vi "Lettura 3 Proximity_fin excel .vi"() -> ()   [LabVIEW 2020]
uses:
  <vilib>/DAQmx/read.llb/DAQmx Read (Analog 1D Wfm NChan NSamp).vi
  <vilib>/Analysis/baseanly.llb/Mean (DBL).vi
  <vilib>/DAQmx/configure/timing.llb/DAQmx Timing (Sample Clock).vi
  <vilib>/DAQmx/miscellaneous.llb/DAQmx Fill In Error Info.vi
  <vilib>/Utility/file.llb/Write Delimited Spreadsheet (DBL).vi
  <vilib>/Analysis/NI_AALBase.lvlib
panel:
  in  "File Excel 3 Sensori":path
  in  "File txt Tensione 1":path
  out "Distanza 1":dbl[](graph)
  in  "File txt Distanza 1":path
  out "Media 3":dbl format="%0.2f"
  out "Deviazione Standard 3":dbl format="%0.2f"
  out "Massimo3":dbl
  out "Minimo 3":dbl
  in  "File txt Tensione 2":path
  out "Distanza 2":dbl[](graph)
  in  "File txt Distanza 2":path
  out "Media 2":dbl format="%0.2f"
  out "Deviazione Standard 2":dbl format="%0.2f"
  out "Massimo 2":dbl
  out "Minimo 2":dbl
  out "Segnale Proximity 1":dynamicdata(graph)
  out "Segnale Proximity 2":dynamicdata(graph)
  out "Minimo":dbl
  out "Massimo":dbl
  out "Deviazione Standard":dbl format="%0.2f"
  out "Media":dbl format="%0.2f"
  in  "File txt Distanza 3":path
  out "Distanza 3":dbl[](graph)
  out "Segnale Proximity 3":dynamicdata(graph)
  out "num campioni":dbl
  in  "File txt Tensione 3":path
  in  "SAVE":bool
  in  "Frequenza":dbl=5000.0 format="%0.2p"
  in  "Durata":dbl=0.1 format="%.2p"
  in  "STOP":bool
  out "current time":timestamp
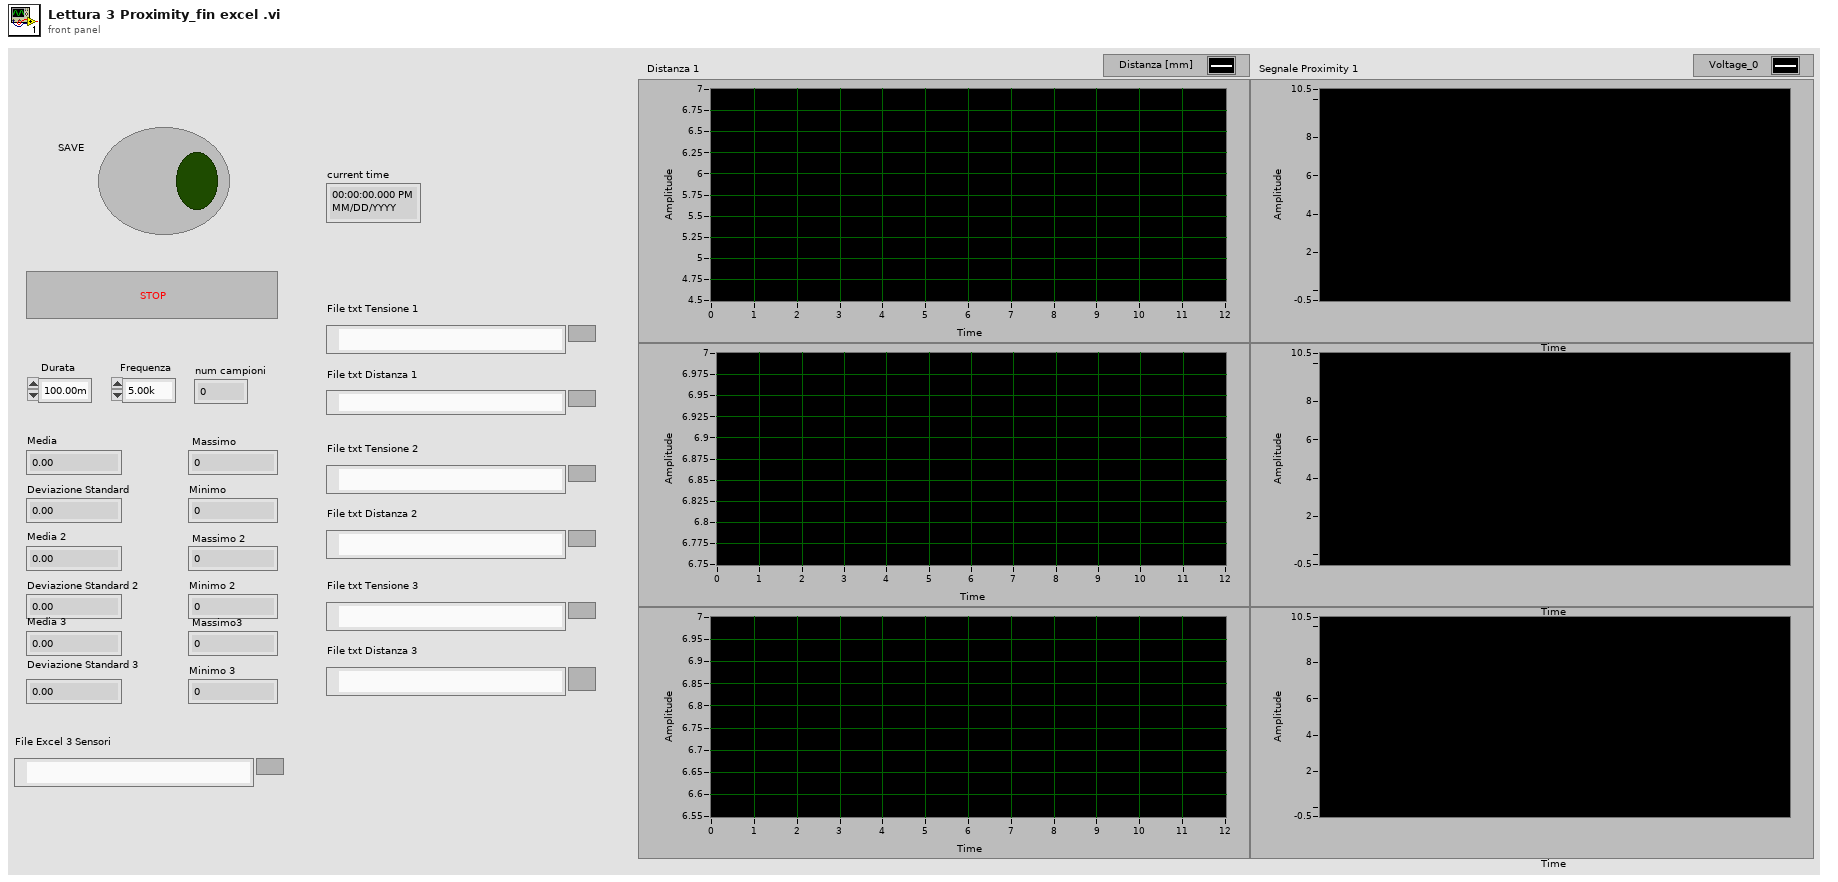
[diagram p1: front panel]
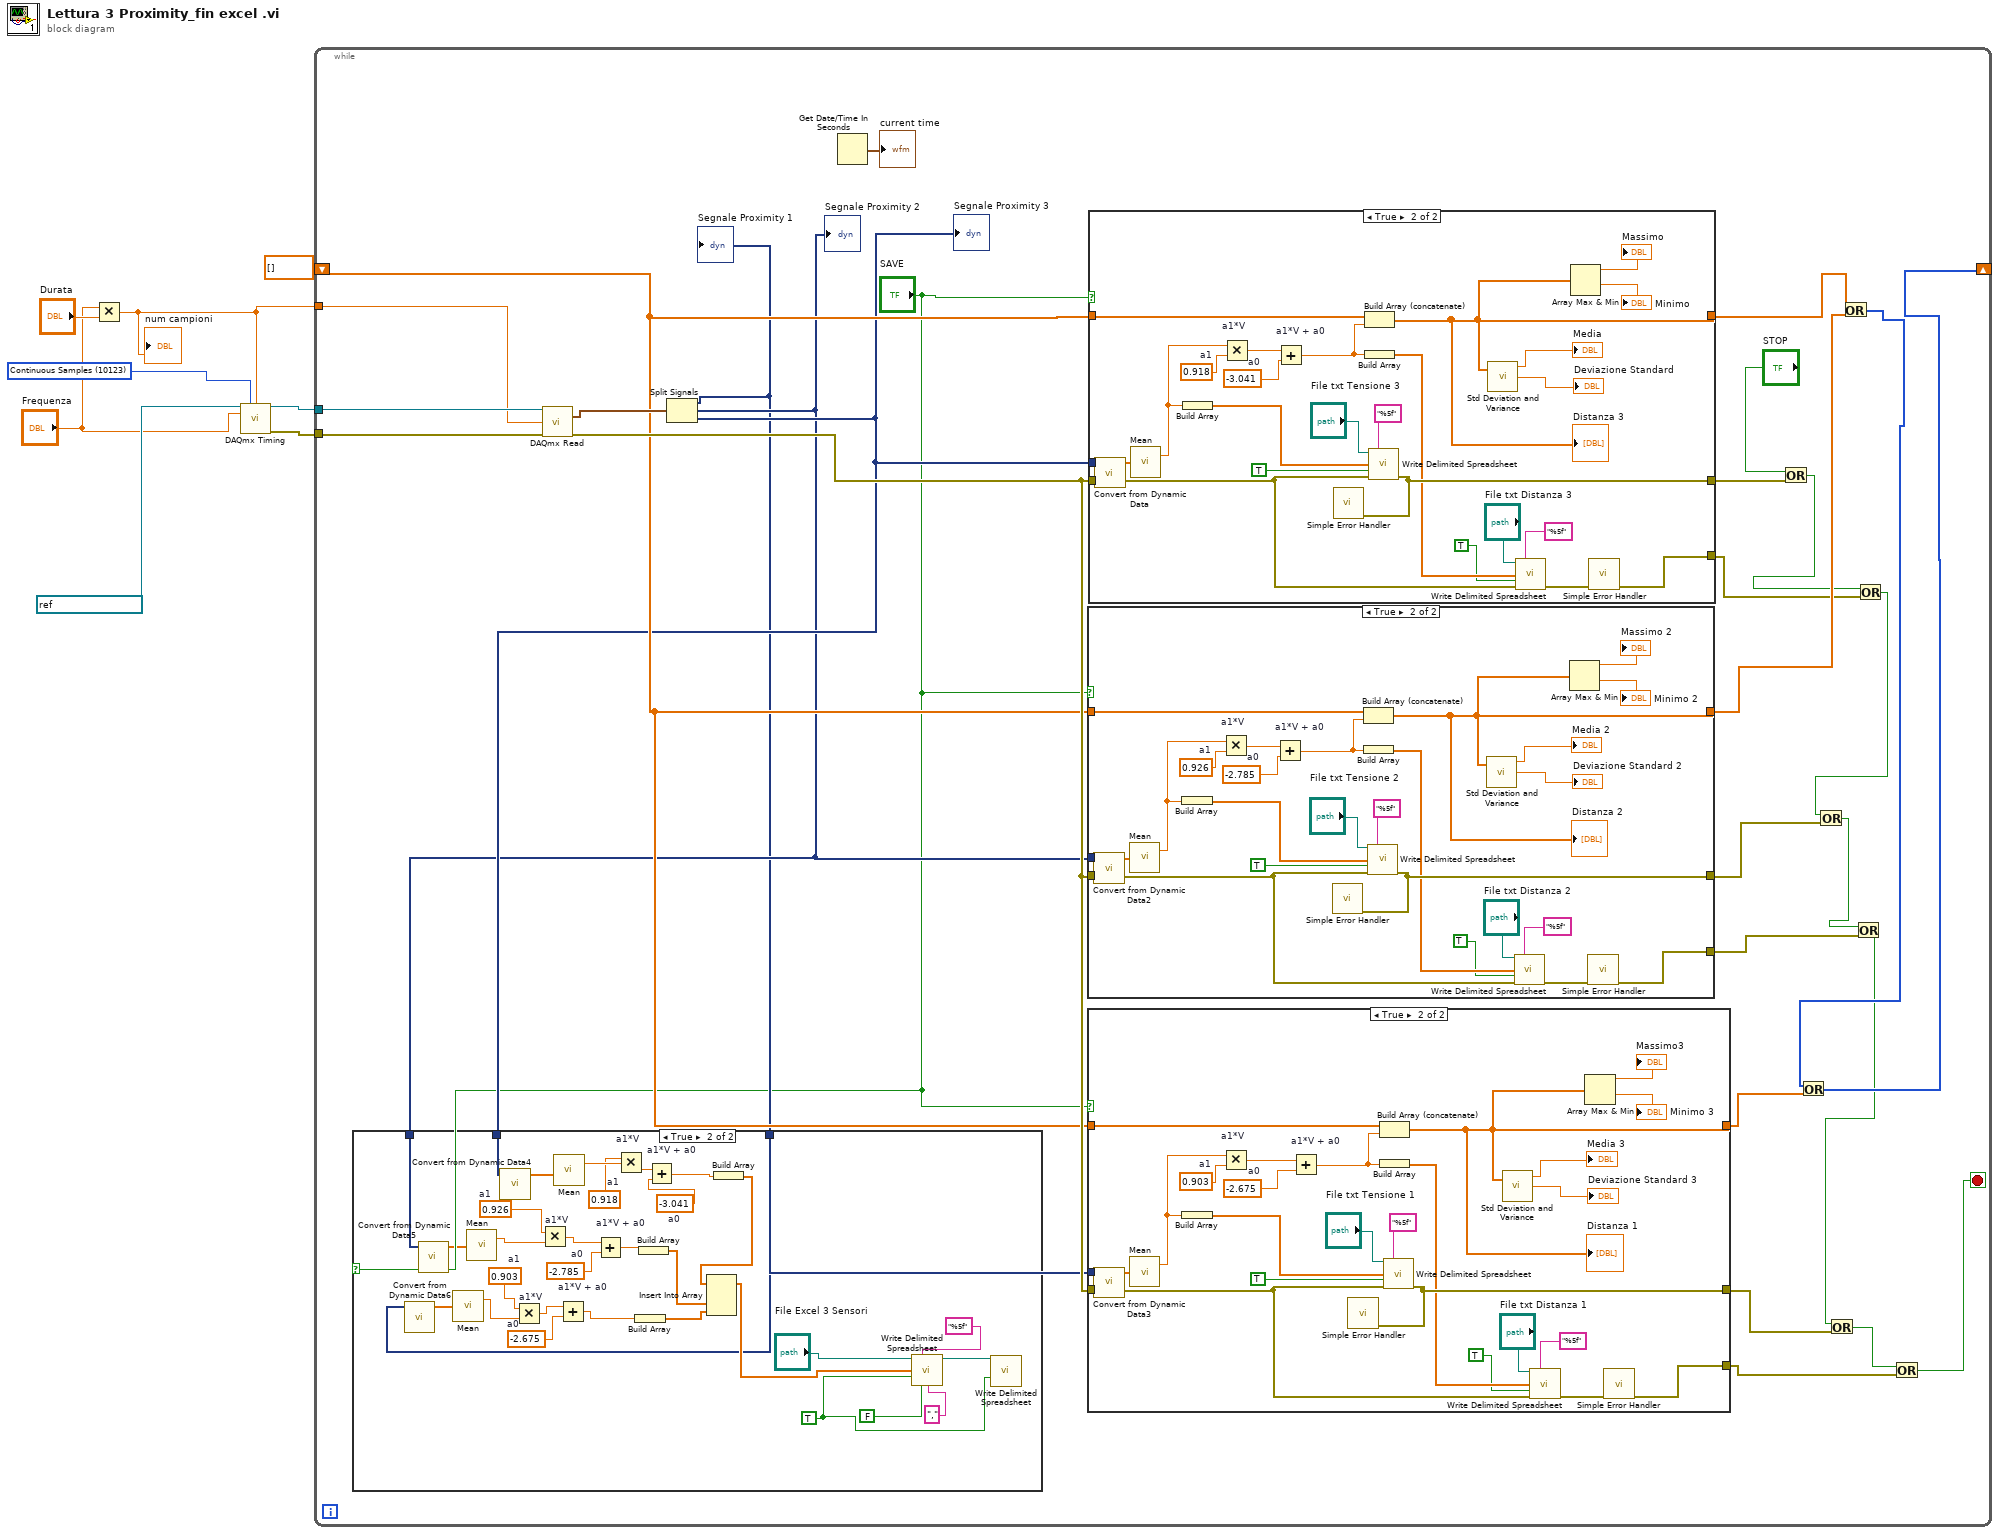
[diagram p0: block diagram]
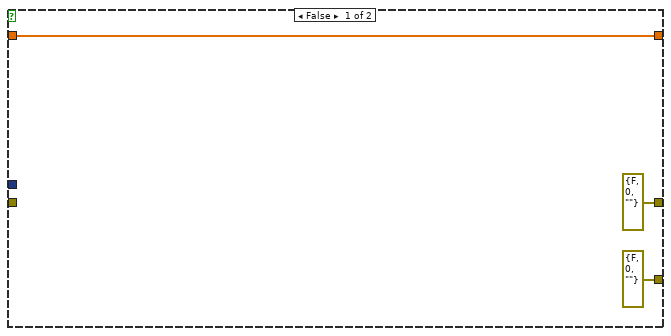
[diagram p3: hidden frame]
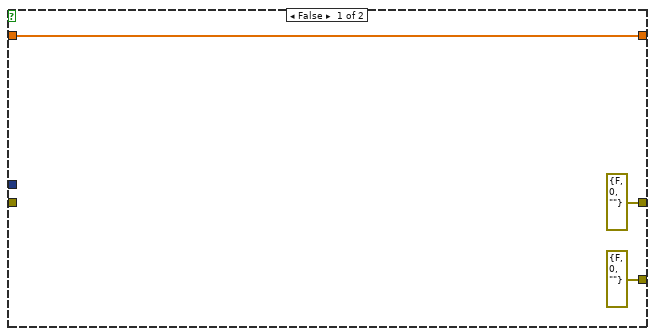
[diagram p4: hidden frame]
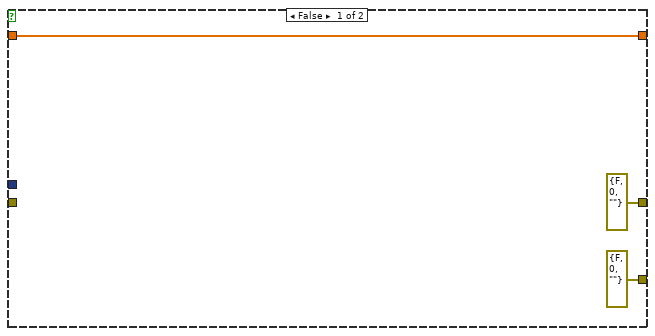
[diagram p5: hidden frame]
diagram:
  w4 = 10123 items=["Finite Samples"=10178, "Continuous Samples"=10123, "Hardware Timed Single Point"=12522] ("sample mode")
  n1 = Multiply(x="Frequenza", y="Durata") -> (x*y=w5:dbl)
  "num campioni" <- w5
  n2 = call-poly <vilib>:"DAQmx Timing.vi"("task/channels in"=refnum<k21> "MyVoltageTask", "sample mode"=w4, "samples per channel"=w5, "rate"="Frequenza") -> ("task out"=w8:refnum<k21>, "error out"=w3:errorcluster)  [unwired: 10 in]
  n3 = while {
    tunnel: w8 -> [w36]
    tunnel: w5 -> [w35]
    tunnel: w3 -> [w34]
    shift-right: [w23] -> _
    shift-left: dbl[] [] -> [w21]
    stop <- w13 stop-if-true
    n4 = call-poly <vilib>:"DAQmx Read.vi"("task/channels in"=w36, "number of samples per channel"=w35, "error in"=w34) -> ("data"=w32:waveform(dbl)[], "error out"=w22:errorcluster)  [unwired: 10 in, 1 out]
    n5 = Split Signals(w32) -> (w10:dynamicdata, w11:dynamicdata, w12:dynamicdata)  [unwired: 3 in]
    "Segnale Proximity 3" <- w12
    "Segnale Proximity 2" <- w11
    "Segnale Proximity 1" <- w10
    n6 = case shown="True" "SAVE" {
      tunnel: w12 -> [_ w63]
      tunnel: w11 -> [_ w54]
      tunnel: w10 -> [_ w62]
      frame False {
      }
      frame True {
        w40 = -2.675  # a0
        w43 = 0.903  # a1
        w41 = -2.785  # a0
        w45 = 0.926  # a1
        w46 = -3.041  # a0
        w47 = 0.918  # a1
        w38 = TRUE ("append to file? (new file:F)")
        n7 = call "Convert from Dynamic Data6"("Dynamic Data Type"=w62) -> ("Array"=w64:dbl[])  [unwired: 3 in]
        n8 = call "Convert from Dynamic Data5"("Dynamic Data Type"=w54) -> ("Array"=w53:dbl[])  [unwired: 3 in]
        n9 = call-poly <vilib>:"Mean.vi"("X"=w64) -> ("mean"=w49:dbl)  [unwired: 1 out]
        n10 = call-poly <vilib>:"Mean.vi"("X"=w53) -> ("mean"=w52:dbl)  [unwired: 1 out]
        n11 = call "Convert from Dynamic Data4"("Dynamic Data Type"=w63) -> ("Array"=w65:dbl[])  [unwired: 3 in]
        n12 = Multiply "a1*V"(x=w43, y=w49) -> (x*y=w44:dbl)
        n13 = Multiply "a1*V"(x=w45, y=w52) -> (x*y=w42:dbl)
        n14 = call-poly <vilib>:"Mean.vi"("X"=w65) -> ("mean"=w55:dbl)  [unwired: 1 out]
        n15 = Add "a1*V + a0"(x=w44, y=w40) -> (x+y=w48:dbl)
        n16 = Add "a1*V + a0"(x=w42, y=w41) -> (x+y=w51:dbl)
        n17 = Multiply "a1*V"(x=w47, y=w55) -> (x*y=w58:dbl)
        n18 = Build Array(w48) -> (w61:dbl[])
        n19 = Build Array(w51) -> (w50:dbl[])
        n20 = Add "a1*V + a0"(x=w58, y=w46) -> (x+y=w57:dbl)
        n21 = Build Array(w57) -> (w56:dbl[])
        n22 = Insert Into Array(array=w56, new element #1=w50, new element #2=w61) -> (w66:dbl[])  [unwired: 1 in]
        n23 = call-poly <vilib>:"Write Delimited Spreadsheet.vi"("file path (dialog if empty)"="File Excel 3 Sensori", "format (%.3f)"="%5f", "1D data"=w66, "append to file? (new file:F)"=w38, "transpose? (no:F)"=FALSE ("append to file? (new file:F)"), "delimiter (\\t)"="," ("format (%.3f)")) -> ("new file path (Not A Path if cancelled)"=w39:path)  [unwired: 8 in, 1 out]
        n24 = call-poly <vilib>:"Write Delimited Spreadsheet.vi"("file path (dialog if empty)"=w39, "append to file? (new file:F)"=w38) -> ()  [unwired: 12 in, 2 out]
      }
    }
    n25 = Get Date/Time In Seconds() -> (seconds since 1Jan1904=→"current time":timestamp)
    n26 = case shown="True" "SAVE" {
      tunnel: [errorcluster {"status"=FALSE, "code"=0, "source"=""} ("error IO") w123] -> w29
      tunnel: w11 -> [_ w122]
      tunnel: w22 -> [_ w115]
      tunnel: [w98 w103] -> w31
      tunnel: w21 -> [w98 w106]
      tunnel: [errorcluster {"status"=FALSE, "code"=0, "source"=""} ("error out") w113] -> w25
      frame False {
      }
      frame True {
        w108 = -2.785  # a0
        w109 = 0.926  # a1
        n27 = call "Convert from Dynamic Data2"("Dynamic Data Type"=w122) -> ("Array"=w100:dbl[])  [unwired: 3 in]
        n28 = call-poly <vilib>:"Mean.vi"("X"=w100) -> ("mean"=w110:dbl)  [unwired: 1 out]
        n29 = Build Array(w110) -> (w119:dbl[])
        n30 = Multiply "a1*V"(x=w110, y=w109) -> (x*y=w111:dbl)
        n31 = Add "a1*V + a0"(x=w111, y=w108) -> (x+y=w107:dbl)
        n32 = Build Array (concatenate)(w106, w107) -> (w103:dbl[])
        "Distanza 2" <- w103
        n33 = Build Array(w107) -> (w118:dbl[])
        n34 = call-poly <vilib>:"Write Delimited Spreadsheet.vi"("file path (dialog if empty)"="File txt Tensione 2", "format (%.3f)"="%5f", "1D data"=w119, "append to file? (new file:F)"=TRUE, "error in (no error)"=w115) -> ("error out"=w123:errorcluster)  [unwired: 9 in, 1 out]
        n35 = call <vilib>:"Simple Error Handler.vi"("error in (no error)"=w123) -> ()  [unwired: 4 in, 5 out]
        n36 = call <vilib>:"Std Deviation and Variance.vi"("X"=w103) -> ("mean"=→"Media 2":dbl, "standard deviation"=→"Deviazione Standard 2":dbl)  [unwired: 1 in, 1 out]
        n37 = call-poly <vilib>:"Write Delimited Spreadsheet.vi"("file path (dialog if empty)"="File txt Distanza 2", "format (%.3f)"="%5f", "1D data"=w118, "append to file? (new file:F)"=TRUE, "error in (no error)"=w115) -> ("error out"=w114:errorcluster)  [unwired: 9 in, 1 out]
        n38 = Array Max & Min(array=w103) -> (max value=→"Massimo 2":dbl, min value=→"Minimo 2":dbl)  [unwired: 2 out]
        n39 = call <vilib>:"Simple Error Handler.vi"("error in (no error)"=w114) -> ("error out"=w113:errorcluster)  [unwired: 4 in, 4 out]
      }
    }
    n40 = case shown="True" "SAVE" {
      tunnel: [errorcluster {"status"=FALSE, "code"=0, "source"=""} ("error IO") w95] -> w28
      tunnel: w10 -> [_ w94]
      tunnel: w22 -> [_ w87]
      tunnel: [w70 w75] -> w26
      tunnel: w21 -> [w70 w78]
      tunnel: [errorcluster {"status"=FALSE, "code"=0, "source"=""} ("error out") w85] -> w27
      frame False {
      }
      frame True {
        w80 = -2.675  # a0
        w81 = 0.903  # a1
        n41 = call "Convert from Dynamic Data3"("Dynamic Data Type"=w94) -> ("Array"=w72:dbl[])  [unwired: 3 in]
        n42 = call-poly <vilib>:"Mean.vi"("X"=w72) -> ("mean"=w82:dbl)  [unwired: 1 out]
        n43 = Build Array(w82) -> (w91:dbl[])
        n44 = Multiply "a1*V"(x=w82, y=w81) -> (x*y=w83:dbl)
        n45 = Add "a1*V + a0"(x=w83, y=w80) -> (x+y=w79:dbl)
        n46 = Build Array (concatenate)(w78, w79) -> (w75:dbl[])
        "Distanza 1" <- w75
        n47 = Build Array(w79) -> (w90:dbl[])
        n48 = call-poly <vilib>:"Write Delimited Spreadsheet.vi"("file path (dialog if empty)"="File txt Tensione 1", "format (%.3f)"="%5f", "1D data"=w91, "append to file? (new file:F)"=TRUE, "error in (no error)"=w87) -> ("error out"=w95:errorcluster)  [unwired: 9 in, 1 out]
        n49 = call <vilib>:"Simple Error Handler.vi"("error in (no error)"=w95) -> ()  [unwired: 4 in, 5 out]
        n50 = call <vilib>:"Std Deviation and Variance.vi"("X"=w75) -> ("mean"=→"Media 3":dbl, "standard deviation"=→"Deviazione Standard 3":dbl)  [unwired: 1 in, 1 out]
        n51 = call-poly <vilib>:"Write Delimited Spreadsheet.vi"("file path (dialog if empty)"="File txt Distanza 1", "format (%.3f)"="%5f", "1D data"=w90, "append to file? (new file:F)"=TRUE, "error in (no error)"=w87) -> ("error out"=w86:errorcluster)  [unwired: 9 in, 1 out]
        n52 = Array Max & Min(array=w75) -> (max value=→"Massimo3":dbl, min value=→"Minimo 3":dbl)  [unwired: 2 out]
        n53 = call <vilib>:"Simple Error Handler.vi"("error in (no error)"=w86) -> ("error out"=w85:errorcluster)  [unwired: 4 in, 4 out]
      }
    }
    n54 = case shown="True" "SAVE" {
      tunnel: [errorcluster {"status"=FALSE, "code"=0, "source"=""} ("error IO") w151] -> w17
      tunnel: w12 -> [_ w150]
      tunnel: w22 -> [_ w143]
      tunnel: [w126 w131] -> w30
      tunnel: w21 -> [w126 w134]
      tunnel: [errorcluster {"status"=FALSE, "code"=0, "source"=""} ("error out") w141] -> w19
      frame False {
      }
      frame True {
        w136 = -3.041  # a0
        w137 = 0.918  # a1
        n55 = call "Convert from Dynamic Data"("Dynamic Data Type"=w150) -> ("Array"=w128:dbl[])  [unwired: 3 in]
        n56 = call-poly <vilib>:"Mean.vi"("X"=w128) -> ("mean"=w138:dbl)  [unwired: 1 out]
        n57 = Build Array(w138) -> (w147:dbl[])
        n58 = Multiply "a1*V"(x=w138, y=w137) -> (x*y=w139:dbl)
        n59 = Add "a1*V + a0"(x=w139, y=w136) -> (x+y=w135:dbl)
        n60 = Build Array (concatenate)(w134, w135) -> (w131:dbl[])
        "Distanza 3" <- w131
        n61 = Build Array(w135) -> (w146:dbl[])
        n62 = call-poly <vilib>:"Write Delimited Spreadsheet.vi"("file path (dialog if empty)"="File txt Tensione 3", "format (%.3f)"="%5f", "1D data"=w147, "append to file? (new file:F)"=TRUE, "error in (no error)"=w143) -> ("error out"=w151:errorcluster)  [unwired: 9 in, 1 out]
        n63 = call <vilib>:"Simple Error Handler.vi"("error in (no error)"=w151) -> ()  [unwired: 4 in, 5 out]
        n64 = call <vilib>:"Std Deviation and Variance.vi"("X"=w131) -> ("mean"=→"Media":dbl, "standard deviation"=→"Deviazione Standard":dbl)  [unwired: 1 in, 1 out]
        n65 = call-poly <vilib>:"Write Delimited Spreadsheet.vi"("file path (dialog if empty)"="File txt Distanza 3", "format (%.3f)"="%5f", "1D data"=w146, "append to file? (new file:F)"=TRUE, "error in (no error)"=w143) -> ("error out"=w142:errorcluster)  [unwired: 9 in, 1 out]
        n66 = Array Max & Min(array=w131) -> (max value=→"Massimo":dbl, min value=→"Minimo":dbl)  [unwired: 2 out]
        n67 = call <vilib>:"Simple Error Handler.vi"("error in (no error)"=w142) -> ("error out"=w141:errorcluster)  [unwired: 4 in, 4 out]
      }
    }
    n68 = Or(x="STOP", y=w17) -> (x .or. y?=w18:bool)
    n69 = Or(x=w30, y=w31) -> (x .or. y?=w24:i32[])
    n70 = Or(x=w24, y=w26) -> (x .or. y?=w23:i32[])
    n71 = Or(x=w18, y=w19) -> (x .or. y?=w15:bool)
    n72 = Or(x=w15, y=w29) -> (x .or. y?=w14:bool)
    n73 = Or(x=w14, y=w25) -> (x .or. y?=w16:bool)
    n74 = Or(x=w16, y=w28) -> (x .or. y?=w20:bool)
    n75 = Or(x=w20, y=w27) -> (x .or. y?=w13:bool)
  }
